vi "Cluster_to_VData.vi"(0 "cluster":variant, 1 "prefix":string) -> (2 "vdata":variant[](array[variant]))   [LabVIEW 2010]
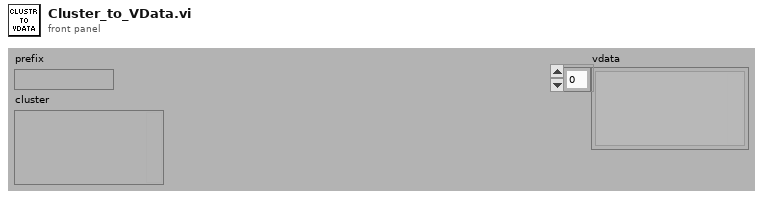
[diagram p1: front panel]
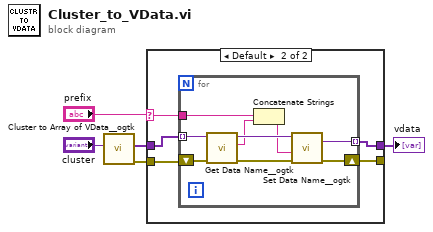
[diagram p0: block diagram]
diagram:
  n1 = call <userlib>:"Cluster to Array of VData__ogtk.vi"("Cluster"="cluster") -> ("error out"=w4:errorcluster, "Array of VData"=w5:variant[])  [unwired: 9 in]
  n2 = case shown="Default" "prefix" {
    selector: "prefix" -> [_ w10]
    tunnel: w5 -> [w7 w12]
    tunnel: w4 -> [w6 w11]
    tunnel: [w7 w9] -> w1
    tunnel: [w6 w8] -> _
    frame "" {
    }
    frame Default {
      n3 = for {
        tunnel: [w19] -> w9 mode=indexing
        tunnel: w12 -> [w18] mode=indexing
        shift-right: [w15] -> w8
        shift-left: w11 -> [w17]
        tunnel: w10 -> [w13]
        n4 = call <userlib>:"Get Data Name__ogtk.vi"("error in (no error)"=w17, "Data"=w18) -> ("error out"=w16:errorcluster, "Data Name"=w14:string, "Data dup"=w21:variant)  [unwired: 7 in]
        n5 = Concatenate Strings(w13, w14) -> (w20:string)
        n6 = call <userlib>:"Set Data Name__ogtk.vi"("error in (no error)"=w16, "Data Name"=w20, "Data"=w21) -> ("error out"=w15:errorcluster, "Renamed Data"=w19:variant)  [unwired: 7 in]
      }
    }
  }
  "vdata" <- w1
